vi "read_N_Dop_relays.vi"() -> (0 "N_Dop Gas Source":bool, 1 "N_Dop H2 Dilute":bool, 2 "N_Dop Remote":bool, 3 "N_Dop Run":bool, 4 "N_Dop Bubbler":bool, 5 "N_Dop Active":bool)   [LabVIEW 2011]
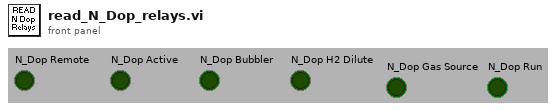
[diagram p1: front panel]
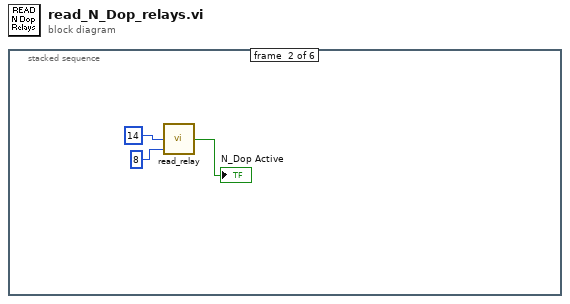
[diagram p0: block diagram]
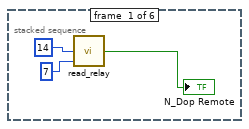
[diagram p2: hidden frame]
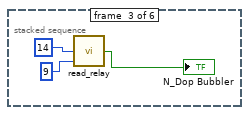
[diagram p3: hidden frame]
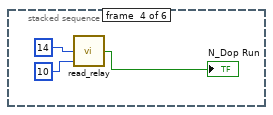
[diagram p4: hidden frame]
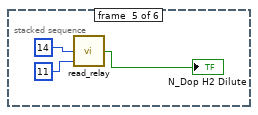
[diagram p5: hidden frame]
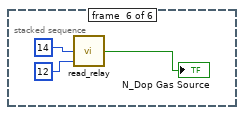
[diagram p6: hidden frame]
diagram:
  n1 = stacked-sequence {
    frame #0 {
      n2 = call "read_relay.vi"("Relay"=7, "Slot"=14) -> ("Relay Status"=→"N_Dop Remote":bool)  [unwired: 1 out]
    }
    frame #1 {
      n3 = call "read_relay.vi"("Relay"=8, "Slot"=14) -> ("Relay Status"=→"N_Dop Active":bool)  [unwired: 1 out]
    }
    frame #2 {
      n4 = call "read_relay.vi"("Relay"=9, "Slot"=14) -> ("Relay Status"=→"N_Dop Bubbler":bool)  [unwired: 1 out]
    }
    frame #3 {
      n5 = call "read_relay.vi"("Relay"=10, "Slot"=14) -> ("Relay Status"=→"N_Dop Run":bool)  [unwired: 1 out]
    }
    frame #4 {
      n6 = call "read_relay.vi"("Relay"=11, "Slot"=14) -> ("Relay Status"=→"N_Dop H2 Dilute":bool)  [unwired: 1 out]
    }
    frame #5 {
      n7 = call "read_relay.vi"("Relay"=12, "Slot"=14) -> ("Relay Status"=→"N_Dop Gas Source":bool)  [unwired: 1 out]
    }
  }
